vi "set parameter - string.vi"(8 "error in (no error)":errorcluster, 9 "value":string, 10 "parameter":u8 format="%x", 11 "channel":u16 format="%x") -> (0 "error out":errorcluster)   [LabVIEW 2024, in "atsj peakcan basic.lvlib"]
doc: "Sets a parameter for a PeakCAN <b>channel</b>."
uses:
  atsj peakcan basic.lvlib
  support/x64/PCANBasic.dll
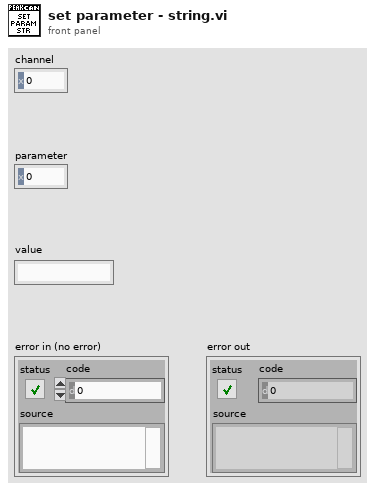
[diagram p1: front panel]
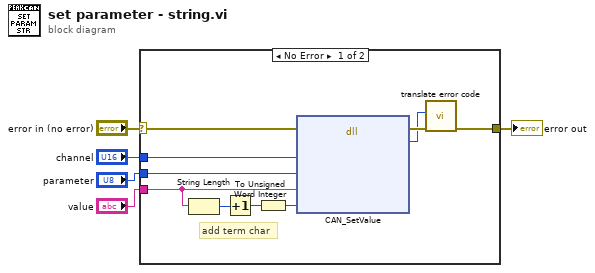
[diagram p0: block diagram]
diagram:
  n1 = case shown="No Error" "error in (no error)" {
    selector: "error in (no error)" -> [w14 w16]
    tunnel: [w15 w16] -> w4
    tunnel: "channel" -> [w11 _]
    tunnel: "parameter" -> [w10 _]
    tunnel: "value" -> [w6 _]
    frame No Error {
      # "add term char"
      n2 = String Length(string=w6) -> (length=w8:i32)
      n3 = Increment(x=w8) -> (x+1=w9:i32)
      n4 = To Unsigned Word Integer(number=w9) -> (unsigned 16bit integer=w7:u16)
      n5 = dll-call lib="C:/atsj/plateau/atsj-peakcan-basic-for-labview/src/support/x64/PCANBasic.dll" fn="CAN_SetValue" ("set parameter - string")(error in=w14, "Channel"=w11, "Parameter"=w10, "Buffer"=w6, "BufferLength"=w7) -> (error out=w13:errorcluster, "Status"=w12:u32)  [unwired: 6 in, 1 out]
      n6 = call "translate error code.vi"("error in (no error)"=w13, "error code"=w12) -> ("error out"=w15:errorcluster)  [unwired: 9 in]
    }
    frame Error {
    }
  }
  "error out" <- w4
